vi "Configure Trigger.vi"(7 "Enable Trigger Delay (Enable)":bool=TRUE, 8 "error in (no error)":errorcluster, 9 "Trigger Delay (0 second)":i32 min=0 max=3600 step=1 format="%#_4f", 10 "Trigger Source (0: Immediate)":u16(ring) format="%.0g" items=["Immediate", "Manual", "External", "Bus"], 11 "VISA resource name":refnum<visa-resource-name>) -> (0 "error out":errorcluster, 3 "VISA resource name out":refnum<visa-resource-name>)   [LabVIEW 2017, in "ADCMT7351_ADC.lvlib"]
doc: "Configures the trigger settings on the instrument.\n\n<B>Note:</B>\nUse this VI only with other low-level VIs. The high-level VIs automatically incorporate this functionality."
uses:
  ADCMT7351_ADC.lvlib
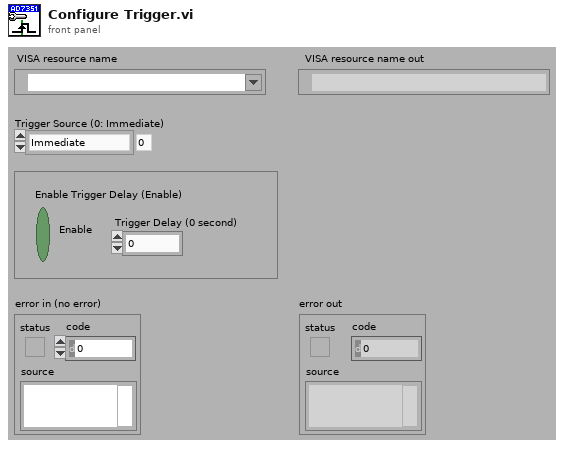
[diagram p1: front panel]
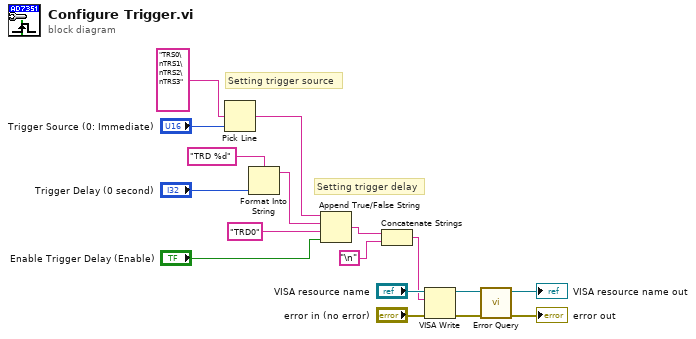
[diagram p0: block diagram]
diagram:
  # "Setting trigger delay"
  # "Setting trigger source"
  n1 = Pick Line(multi-line string="TRS0\nTRS1\nTRS2\nTRS3", line index="Trigger Source (0: Immediate)") -> (output string=w7:string)  [unwired: 1 in]
  n2 = Format Into String(format string="TRD %d" ("Trigger Delay Time Set"), "Trigger Delay (0 second)") -> (resulting string=w6:string)  [unwired: 2 in, 1 out]
  n3 = Append True/False String(1:"Enable Trigger Delay (Enable)", 2:"TRD0" ("Disable Trigger Delay"), 3:w6, 4:w7) -> (0:w3:string)
  n4 = Concatenate Strings(w3, "\n") -> (w1:string)
  n5 = VISA Write(VISA resource name="VISA resource name", write buffer=w1, error in (no error)="error in (no error)") -> (VISA resource name out=w12:refnum<visa-resource-name>, error out=w11:errorcluster)  [unwired: 1 out]
  n6 = call "Error Query.vi"("error in (no error)"=w11, "VISA resource name"=w12) -> ("error out"=→"error out":errorcluster, "VISA resource name out"=→"VISA resource name out":refnum<visa-resource-name>)  [unwired: 6 in, 2 out]
